vi "VIrefParse.vi"(3 "Params":T1, 4 "VIA":string, 5 "String in":string) -> (1 "defaults":string, 2 "String out":string)   [LabVIEW 2014]
panel:
  out "Array":string[](array[string])
  out "Array 2":T2(array[cluster])
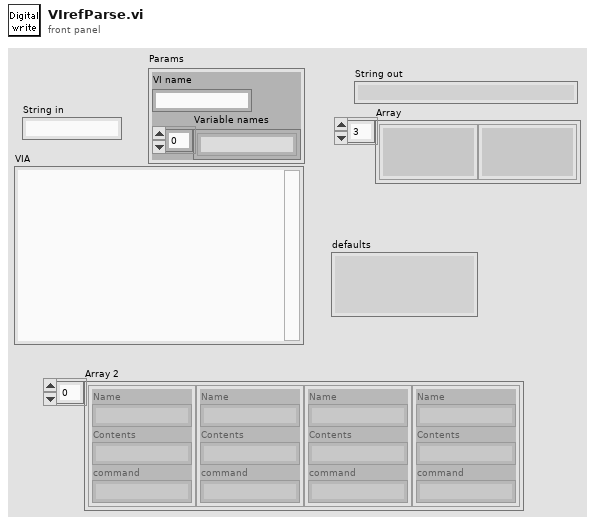
[diagram p1: front panel]
types:
  T1 = cluster{"VI name":string, "Variable names":string[]}
  T2 = cluster{"Name":string, "Contents":string, "command":string}[]
  T3 = cluster{"trimmed string":string, "Contents":string, "command":string}
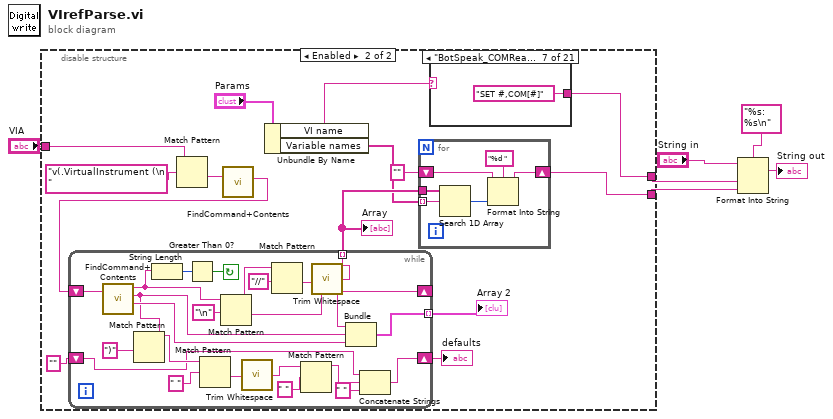
[diagram p0: block diagram]
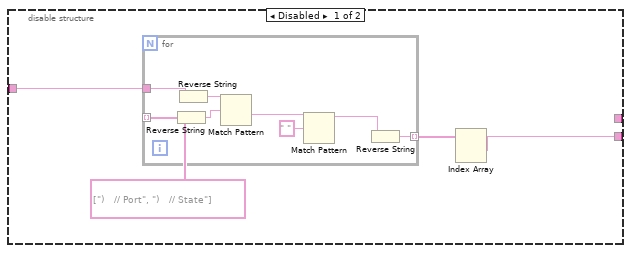
[diagram p2: hidden frame]
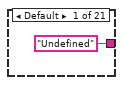
[diagram p3: hidden frame]
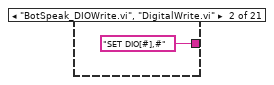
[diagram p4: hidden frame]
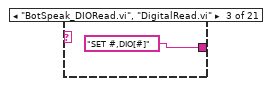
[diagram p5: hidden frame]
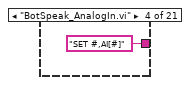
[diagram p6: hidden frame]
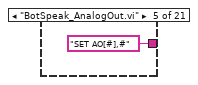
[diagram p7: hidden frame]
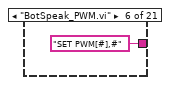
[diagram p8: hidden frame]
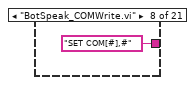
[diagram p9: hidden frame]
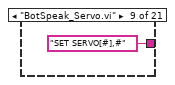
[diagram p10: hidden frame]
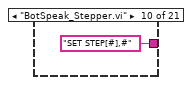
[diagram p11: hidden frame]
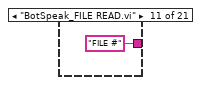
[diagram p12: hidden frame]
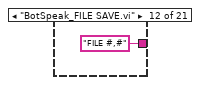
[diagram p13: hidden frame]
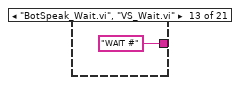
[diagram p14: hidden frame]
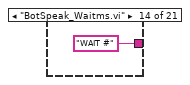
[diagram p15: hidden frame]
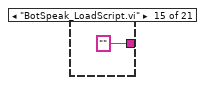
[diagram p16: hidden frame]
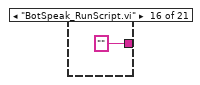
[diagram p17: hidden frame]
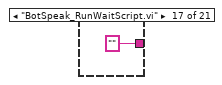
[diagram p18: hidden frame]
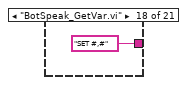
[diagram p19: hidden frame]
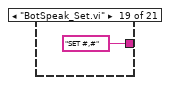
[diagram p20: hidden frame]
diagram:
  n1 = disable-structure shown="Enabled" {
    disable-tunnel: "VIA" -> [w11 w32]
    disable-tunnel: [w8 w25] -> w2
    disable-tunnel: [_ w23] -> w1
    frame Disabled {
      n2 = for {
        tunnel: w11 -> [w19]
        tunnel: [w14] -> w9 mode=indexing
        tunnel: string[] [")   // Port", ")   // State"] -> [w12] mode=indexing
        n3 = Reverse String(1:w12) -> (0:w17:string)
        n4 = Reverse String(1:w19) -> (0:w18:string)
        n5 = Match Pattern(string=w18, regular expression=w17) -> (after substring=w15:string)  [unwired: 1 in, 3 out]
        n6 = Match Pattern(string=w15, regular expression=" ") -> (before substring=w13:string)  [unwired: 1 in, 3 out]
        n7 = Reverse String(1:w13) -> (0:w14:string)
      }
      n8 = Index Array(array=w9) -> (element #1=w8:string, element #2=w7:string)  [unwired: 2 in]
    }
    frame Enabled {
      n9 = Match Pattern(string=w32, regular expression="v(.VirtualInstrument (\n   ") -> (after substring=w31:string)  [unwired: 1 in, 3 out]
      n10 = call <vilib>:"FindCommand+Contents.vi"("Via file in"=w31) -> ("Contents"=w30:string)  [unwired: 1 in, 3 out]
      n11 = while {
        shift-right: [w77] -> _
        shift-left: w30 -> [w83]
        tunnel: [w79] -> w22 mode=indexing
        tunnel: [w72] -> w29 mode=indexing
        shift-right: [w62] -> w20
        shift-left: "" -> [w64]
        stop <- w81 continue-if-true
        n12 = call <vilib>:"FindCommand+Contents.vi"("Via file in"=w83) -> ("left"=w76:string, "Contents"=w65:string, "command"=w80:string)  [unwired: 1 in, 1 out]
        n13 = Match Pattern(string=w65, regular expression=")") -> (before substring=w70:string)  [unwired: 1 in, 3 out]
        n14 = String Length(string=w76) -> (length=w82:i32)
        n15 = Greater Than 0?(x=w82) -> (x > 0?=w81:bool)
        n16 = Match Pattern(string=w70, regular expression=" ") -> (after substring=w68:string)  [unwired: 1 in, 3 out]
        n17 = Match Pattern(string=w76, regular expression="\n") -> (before substring=w75:string, after substring=w77:string)  [unwired: 1 in, 2 out]
        n18 = call <vilib>:"Trim Whitespace.vi"("string"=w68) -> ("trimmed string"=w67:string)  [unwired: 1 in]
        n19 = Match Pattern(string=w75, regular expression="//") -> (after substring=w74:string)  [unwired: 1 in, 3 out]
        n20 = Match Pattern(string=w67, regular expression=" ") -> (before substring=w63:string)  [unwired: 1 in, 3 out]
        n21 = call <vilib>:"Trim Whitespace.vi"("string"=w74) -> ("trimmed string"=w72:string)  [unwired: 1 in]
        n22 = Bundle("trimmed string"=w72, "Contents"=w65, "command"=w80) -> (w79:T3)  [unwired: 1 in]
        n23 = Concatenate Strings(w64, w63, " " ("string")) -> (w62:string)
      }
      "Array 2" <- w22
      "Array" <- w29
      "defaults" <- w20
      n24 = Unbundle By Name("Params") -> ("VI name"=w24:string, "Variable names"=w27:string[])
      n25 = for {
        tunnel: w27 -> [w60] mode=indexing
        tunnel: w29 -> [w58]
        shift-right: [w56] -> w25
        shift-left: "" -> [w55]
        n26 = Search 1D Array(1D array=w58, element=w60) -> (index of element=w59:i32)  [unwired: 1 in]
        n27 = Format Into String(format string="%d ", initial string=w55, w59) -> (resulting string=w56:string)  [unwired: 1 in, 1 out]
      }
      n28 = case shown="\"BotSpeak_COMRead.vi\"" w24 {
        tunnel: ["Undefined" ("format string") "SET DIO[#],#" ("format string") "SET #,DIO[#]" ("format string") "SET #,AI[#]" ("format string") "SET AO[#],#" ("format string") "SET PWM[#],#" ("format string") "SET #,COM[#]" ("format string") "SET COM[#],#" ("format string") "SET SERVO[#],#" ("format string") "SET STEP[#],#" ("format string") "FILE #" ("format string") "FILE #,#" ("format string") "WAIT #" ("format string") "WAIT #" ("format string") "" ("format string") "" ("format string") "" ("format string") "SET #,#" ("format string") "SET #,#" ("format string") "SET #,VER" ("format string") "SYSTEM #,#" ("format string")] -> w23
        frame Default {
        }
        frame "BotSpeak_DIOWrite.vi", "DigitalWrite.vi" {
        }
        frame "BotSpeak_DIORead.vi", "DigitalRead.vi" {
        }
        frame "BotSpeak_AnalogIn.vi" {
        }
        frame "BotSpeak_AnalogOut.vi" {
        }
        frame "BotSpeak_PWM.vi" {
        }
        frame "BotSpeak_COMRead.vi" {
        }
        frame "BotSpeak_COMWrite.vi" {
        }
        frame "BotSpeak_Servo.vi" {
        }
        frame "BotSpeak_Stepper.vi" {
        }
        frame "BotSpeak_FILE READ.vi" {
        }
        frame "BotSpeak_FILE SAVE.vi" {
        }
        frame "BotSpeak_Wait.vi", "VS_Wait.vi" {
        }
        frame "BotSpeak_Waitms.vi" {
        }
        frame "BotSpeak_LoadScript.vi" {
        }
        frame "BotSpeak_RunScript.vi" {
        }
        frame "BotSpeak_RunWaitScript.vi" {
        }
        frame "BotSpeak_GetVar.vi" {
        }
        frame "BotSpeak_Set.vi" {
        }
        frame "BotSpeak_GetVer.vi" {
        }
        frame "BotSpeak_System.vi" {
        }
      }
    }
  }
  n29 = Format Into String(format string="%s: %s\n" ("regular expression"), initial string="String in", w1, w2) -> (resulting string=→"String out":string)  [unwired: 1 in, 1 out]
